vi "XBox-Set Mouse Wheel Window.vi"(0 "VI ref":refnum<vi>, 11 "error in (no error)":errorcluster) -> (8 "ScrollWheelValue":i32, 15 "error out":errorcluster)   [LabVIEW 2015]
uses:
  D:/Experiment VIs/Utility VIs/Windows VIs/WindowWrapper.dll
  Windows VIs/WindowWrapper.dll
  Microsoft.Xna.Framework
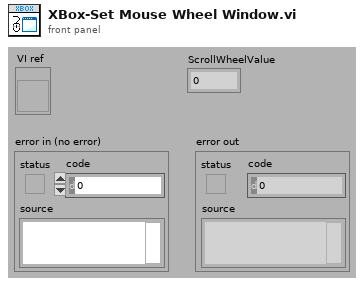
[diagram p1: front panel]
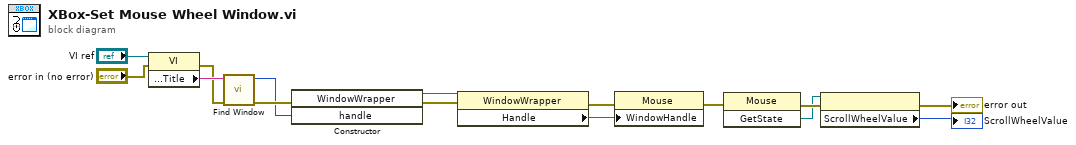
[diagram p0: block diagram]
diagram:
  n1 = property class="VI"(reference="VI ref", error in="error in (no error)") -> (error out=w12:errorcluster, "Front Panel.Title"=w15:string)  [unwired: 1 out]
  n2 = call "Find Window.vi"("error in (no error)"=w12, "Window Name"=w15) -> ("error out"=w11:errorcluster, "Win32 Window Handle"=w10:i32)  [unwired: 8 in]
  n3 = constructor class="WindowWrapper"(error in=w11, "handle"=w10) -> (reference out=w9:refnum<k24>, error out=w8:errorcluster)  [unwired: 2 in, 2 out]
  n4 = property class="WindowWrapper"(reference=w9, error in=w8) -> (error out=w6:errorcluster, "Handle"=w7:refnum<k24>)  [unwired: 1 out]
  n5 = property class="Mouse"(error in=w6, "WindowHandle"=w7) -> (error out=w3:errorcluster)  [unwired: 1 in, 1 out]
  n6 = invoke class="Mouse" method="GetState"(error in=w3) -> (error out=w5:errorcluster, "GetState"=w4:refnum<k24>)  [unwired: 2 in, 1 out]
  n7 = property(reference=w4, error in=w5) -> (error out=→"error out":errorcluster, "ScrollWheelValue"=→"ScrollWheelValue":i32)  [unwired: 1 out]
